vi "_ADC Calibration.vi"(0 "ADC In":string[][](table)) -> (1 "ADC Out":string[][](table), 2 "ADC Table":T1[](array[typedef]))   [LabVIEW 2012]
uses:
  Type/_RT Configuration 2.ctl
  Type/_RT Command.ctl
  Type/_RT Active Ch.ctl
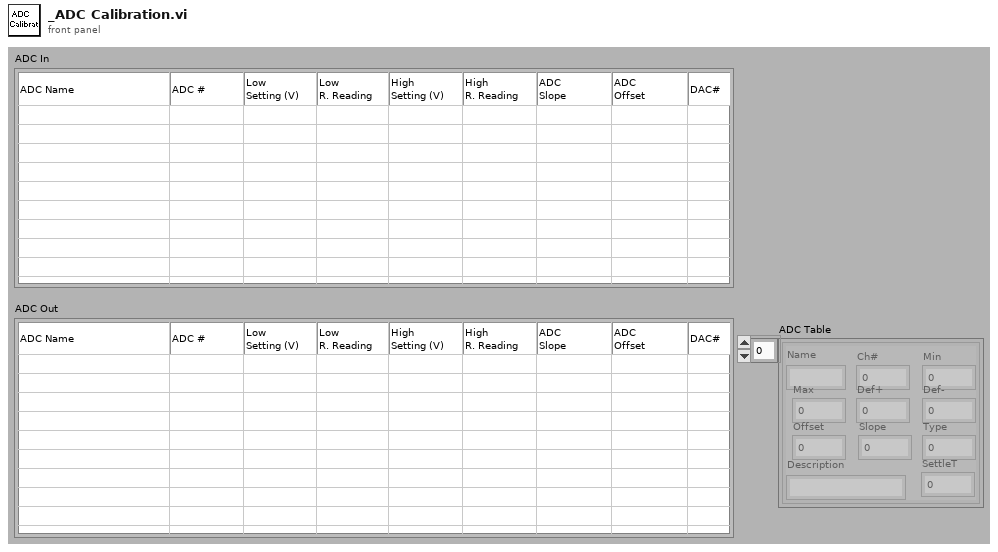
[diagram p1: front panel]
types:
  T1 = typedef "_RT Configuration 2.ctl" = cluster{"Name":string, "Ch#":u8, "Min":dbl, "Max":dbl, "Def+":dbl, "Def-":dbl, "Offset":dbl, "Slope":dbl, "Type":u8, "Description":string, "SettleT":dbl}
  T2 = typedef "_RT Command.ctl" = enum16{"Start", "Stop", "Runtime Update", "Get Data", "Get Info", "Get Status", "Get Param", "Get Config", "Get Table", "Read ADC", "Set Oscillator", "Update Config", "Update Table", "Set All Pol", "Set Pol and DC", "Set Max Mass", "Toggle RP", "Toggle EL", "Set PIC", "Initialize Turbo", "Send Turbo Comm", "Close Turbo", "P1", "P2", "P3", "Send Serial", "Set LC Out", "Get LC In", "Read VAC", "Test Table", "Toggle Power", "Get Startup", "Set Startup", "Get ADC Table", "Set ADC Table", "Get Brief Status", "Get Detail Status", "Auxiliary Update", "Set CC Logics", "Set CC Input Logics", "Ignore Error"}
  T3 = typedef "_RT Active Ch.ctl" = cluster{"Start":i32, "Step":i32, "ChID":i32}
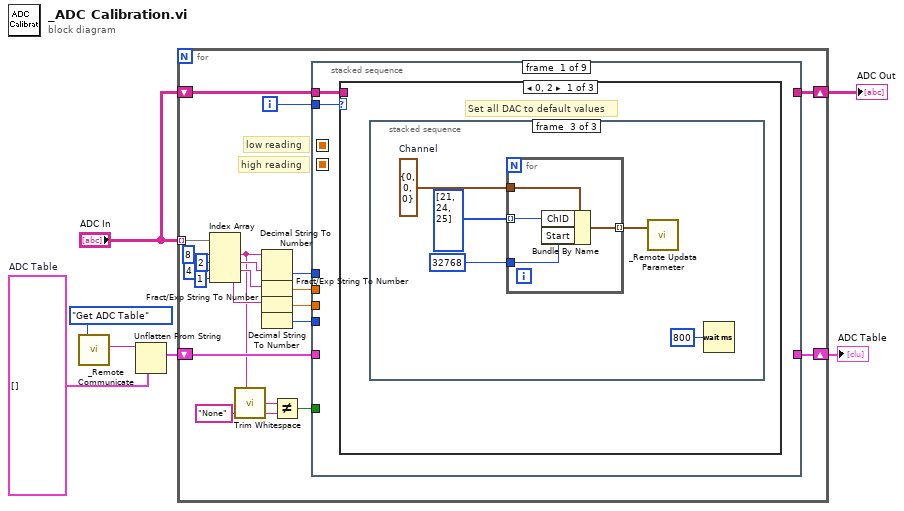
[diagram p0: block diagram]
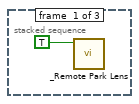
[diagram p2: hidden frame]
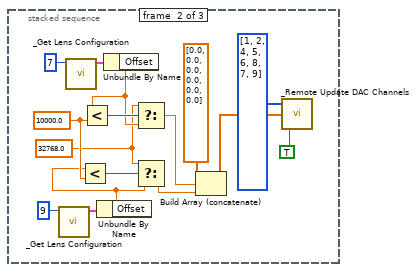
[diagram p3: hidden frame]
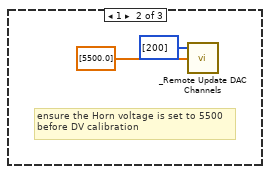
[diagram p4: hidden frame]
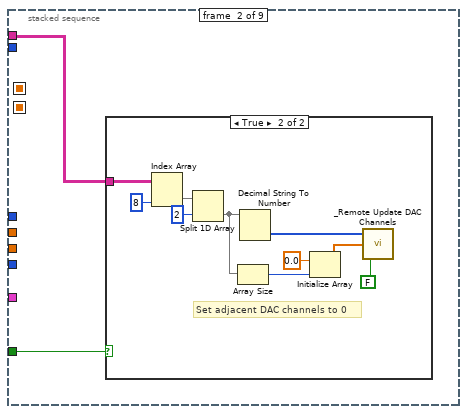
[diagram p6: hidden frame]
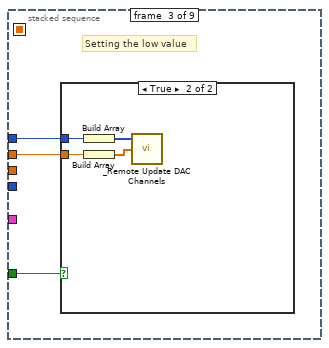
[diagram p8: hidden frame]
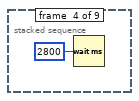
[diagram p10: hidden frame]
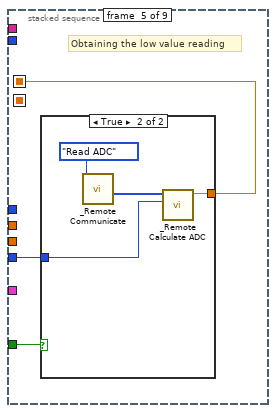
[diagram p11: hidden frame]
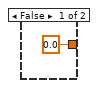
[diagram p12: hidden frame]
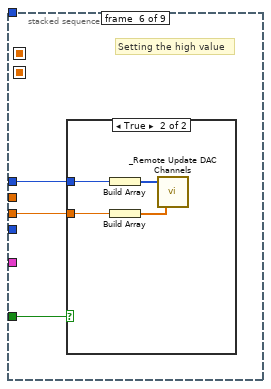
[diagram p13: hidden frame]
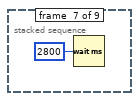
[diagram p15: hidden frame]
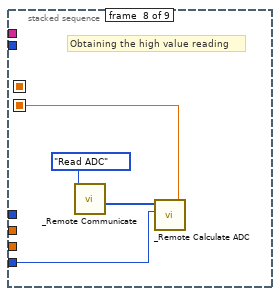
[diagram p16: hidden frame]
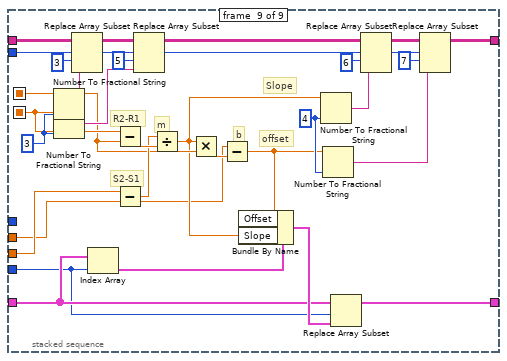
[diagram p17: hidden frame]
diagram:
  w3 = T1[] []  # ADC Table
  n1 = call "_Remote Communicate.vi"("Command"=_RT_Command."Get ADC Table") -> ("Info"=w4:string)  [unwired: 5 in, 3 out]
  n2 = Unflatten From String(type=w3, binary string=w4) -> (value=w2:T1[])  [unwired: 1 in, 4 out]
  n3 = for {
    tunnel: "ADC In" -> [w28] mode=indexing
    shift-right: [w22] -> w6
    shift-left: "ADC In" -> [w23]
    shift-right: [w12] -> w1
    shift-left: w2 -> [w21]
    i -> [w26]
    # "high reading"
    # "low reading"
    n4 = Index Array(array=w28, index #1=8 ("index"), index #2=2 ("index"), index #3=4 ("index"), index #4=1 ("index")) -> (element #1=w9:string, element #2=w19:string, element #3=w16:string, element #4=w14:string)
    n5 = call <vilib>:"Trim Whitespace.vi"("string"=w9) -> ("trimmed string"=w11:string)  [unwired: 1 in]
    n6 = Decimal String To Number(string=w9) -> (number=w27:i32)  [unwired: 3 out]
    n7 = Fract/Exp String To Number(string=w19) -> (number=w25:dbl)  [unwired: 4 out]
    n8 = Fract/Exp String To Number(string=w16) -> (number=w24:dbl)  [unwired: 4 out]
    n9 = Decimal String To Number(string=w14) -> (number=w13:i32)  [unwired: 3 out]
    n10 = Not Equal?(x=w11, y="None") -> (x != y?=w8:bool)
    n11 = stacked-sequence {
      seq-local: [_ _ _ _ w80 _ _ _ _] -> [_ _ _ _ _ _ _ _ w107]
      seq-local: [_ _ _ _ _ _ _ w95 _] -> [_ _ _ _ _ _ _ _ w111]
      tunnel: w27 -> [_ _ w73 _ _ w89 _ _ _]
      tunnel: w26 -> [w30 _ _ _ _ _ _ _ w115]
      tunnel: w25 -> [_ _ w72 _ _ _ _ _ w104]
      tunnel: w24 -> [_ _ _ _ _ w88 _ _ w110]
      tunnel: w23 -> [w29 w60 _ _ _ _ _ _ w117]
      tunnel: [_ _ _ _ _ _ _ _ w121] -> w22
      tunnel: w21 -> [_ _ _ _ _ _ _ _ w101]
      tunnel: w13 -> [_ _ _ _ w81 _ _ w96 w99]
      tunnel: [_ _ _ _ _ _ _ _ w100] -> w12
      tunnel: w8 -> [_ w59 w71 _ w79 w87 _ _ _]
      frame #0 {
        n12 = case shown="0, 2" w30 {
          tunnel: w29 -> [_ _ _]
          frame 0, 2 {
            # "Set all DAC to default values"
            n13 = stacked-sequence {
              frame #0 {
                n14 = call "_Remote Park Lens.vi"("All Ch (F)"=TRUE) -> ()  [unwired: 1 in, 6 out]
              }
              frame #1 {
                w36 = 32768.0 ("y")
                w38 = 10000.0 ("y")
                n15 = call "_Get Lens Configuration.vi"("Channel #"=u8 9) -> ("Lens Configuration"=w43:T1)  [unwired: 1 in, 5 out]
                n16 = call "_Get Lens Configuration.vi"("Channel #"=u8 7) -> ("Lens Configuration"=w44:T1)  [unwired: 1 in, 5 out]
                n17 = Unbundle By Name(w43) -> ("Offset"=w37:dbl)
                n18 = Less?(x=w37, y=w38) -> (x < y?=w39:bool)
                n19 = Unbundle By Name(w44) -> ("Offset"=w40:dbl)
                n20 = Less?(x=w40, y=w38) -> (x < y?=w41:bool)
                n21 = Select(t=w36, s=w41, f=w40) -> (s? t:f=w33:dbl)
                n22 = Select(t=w36, s=w39, f=w37) -> (s? t:f=w32:dbl)
                n23 = Build Array (concatenate)(dbl[] [0.0, 0.0, 0.0, 0.0, 0.0, 0.0] ("Ch#"), w33, w32) -> (w34:dbl[])
                n24 = call "_Remote Update DAC Channels.vi"("In DAC(F)"=TRUE ("Zero-DAC (F)"), "UserValue"=w34, "Ch#"=u8[] [1, 2, 4, 5, 6, 8, 7, 9]) -> ()  [unwired: 2 out]
              }
              frame #2 {
                w49 = T3 {"Start"=0, "Step"=0, "ChID"=0}  # Channel
                n25 = for {
                  tunnel: u8[] [21, 24, 25] ("Ch#") -> [w56] mode=indexing
                  tunnel: 32768 ("Start") -> [w55]
                  tunnel: w49 -> [w54]
                  tunnel: [w53] -> w48 mode=indexing
                  n26 = Bundle By Name(cluster=w54, "ChID"=w56, "Start"=w55) -> (w53:T3)
                }
                n27 = call "_Remote Updata Parameter.vi"("Parameters"=w48) -> ()  [unwired: 1 in, 1 out]
                n28 = Wait (ms)(milliseconds to wait=u32 800) -> ()  [unwired: 1 out]
              }
            }
          }
          frame 1 {
            # "ensure the Horn voltage is set to 5500\nbefore DV calibration"
            n29 = call "_Remote Update DAC Channels.vi"("UserValue"=dbl[] [5500.0], "Ch#"=i32[] [200]) -> ()  [unwired: 1 in, 2 out]
          }
          frame Default {
          }
        }
      }
      frame #1 {
        n30 = case shown="True" w59 {
          tunnel: w60 -> [_ w61]
          frame False {
          }
          frame True {
            # "Set adjacent DAC channels to 0"
            n31 = Index Array(array=w61, index (col)=8 ("disabled index (col)")) -> (element=w69:string[])  [unwired: 1 in]
            n32 = Split 1D Array(array=w69, index=2) -> (second subarray=w67:string[])  [unwired: 1 out]
            n33 = Array Size(array=w67) -> (size(s)=w66:i32)
            n34 = Decimal String To Number(string=w67) -> (number=w63:i32[])  [unwired: 3 out]
            n35 = Initialize Array(0.0 ("element"), w66) -> (w62:dbl[])
            n36 = call "_Remote Update DAC Channels.vi"("In DAC(F)"=FALSE ("Zero-DAC (F)"), "UserValue"=w62, "Ch#"=w63) -> ()  [unwired: 2 out]
          }
        }
      }
      frame #2 {
        # "Setting the low value"
        n37 = case shown="True" w71 {
          tunnel: w73 -> [_ w77]
          tunnel: w72 -> [_ w75]
          frame False {
          }
          frame True {
            n38 = Build Array(w77) -> (w76:i32[])
            n39 = Build Array(w75) -> (w74:dbl[])
            n40 = call "_Remote Update DAC Channels.vi"("UserValue"=w74, "Ch#"=w76) -> ()  [unwired: 1 in, 2 out]
          }
        }
      }
      frame #3 {
        n41 = Wait (ms)(milliseconds to wait=u32 2800) -> ()  [unwired: 1 out]
      }
      frame #4 {
        # "Obtaining the low value reading"
        n42 = case shown="True" w79 {
          tunnel: w81 -> [_ w84]
          tunnel: [0.0 ("Raw Reading") w83] -> w80
          frame False {
          }
          frame True {
            n43 = call "_Remote Communicate.vi"("Command"=_RT_Command."Read ADC") -> ("Data Array"=w85:i32[])  [unwired: 5 in, 3 out]
            n44 = call "_Remote Calculate ADC.vi"("ADC Channel (64)"=w84, "ADC Values"=w85) -> ("Raw Reading"=w83:dbl)  [unwired: 2 in, 3 out]
          }
        }
      }
      frame #5 {
        # "Setting the high value"
        n45 = case shown="True" w87 {
          tunnel: w89 -> [_ w93]
          tunnel: w88 -> [_ w90]
          frame False {
          }
          frame True {
            n46 = Build Array(w93) -> (w92:i32[])
            n47 = Build Array(w90) -> (w91:dbl[])
            n48 = call "_Remote Update DAC Channels.vi"("UserValue"=w91, "Ch#"=w92) -> ()  [unwired: 1 in, 2 out]
          }
        }
      }
      frame #6 {
        n49 = Wait (ms)(milliseconds to wait=u32 2800) -> ()  [unwired: 1 out]
      }
      frame #7 {
        # "Obtaining the high value reading"
        n50 = call "_Remote Communicate.vi"("Command"=_RT_Command."Read ADC") -> ("Data Array"=w97:i32[])  [unwired: 5 in, 3 out]
        n51 = call "_Remote Calculate ADC.vi"("ADC Channel (64)"=w96, "ADC Values"=w97) -> ("Raw Reading"=w95:dbl)  [unwired: 2 in, 3 out]
      }
      frame #8 {
        w114 = i16 3 ("precision (6)")
        w127 = i16 4 ("precision (6)")
        # "Slope"
        # "b"
        # "offset"
        # "m"
        # "S2-S1"
        # "R2-R1"
        n52 = Number To Fractional String(number=w107, precision (6)=w114) -> (F-format string=w113:string)  [unwired: 2 out]
        n53 = Number To Fractional String(number=w111, precision (6)=w114) -> (F-format string=w112:string)  [unwired: 2 out]
        n54 = Replace Array Subset(array=w117, new element=w113, index (row)=w115, index (col)=3 ("disabled index (col)")) -> (w120:string[][])
        n55 = Index Array(array=w101, index=w99) -> (element=w102:T1)
        n56 = Subtract(x=w111, y=w107) -> (x-y=w109:dbl)
        n57 = Subtract(x=w110, y=w104) -> (x-y=w108:dbl)
        n58 = Replace Array Subset(array=w120, new element=w112, index (row)=w115, index (col)=5 ("disabled index (col)")) -> (w116:string[][])
        n59 = Divide(x=w108, y=w109) -> (x/y=w106:dbl)
        n60 = Multiply(x=w106, y=w107) -> (x*y=w105:dbl)
        n61 = Subtract(x=w104, y=w105) -> (x-y=w103:dbl)
        n62 = Bundle By Name(cluster=w102, "Offset"=w103, "Slope"=w106) -> (w128:T1)
        n63 = Number To Fractional String(number=w106, precision (6)=w127) -> (F-format string=w125:string)  [unwired: 2 out]
        n64 = Number To Fractional String(number=w103, precision (6)=w127) -> (F-format string=w122:string)  [unwired: 2 out]
        n65 = Replace Array Subset(array=w101, new element=w128, index=w99) -> (w100:T1[])
        n66 = Replace Array Subset(array=w116, new element=w125, index (row)=w115, index (col)=6 ("disabled index (col)")) -> (w123:string[][])
        n67 = Replace Array Subset(array=w123, new element=w122, index (row)=w115, index (col)=7 ("disabled index (col)")) -> (w121:string[][])
      }
    }
  }
  "ADC Out" <- w6
  "ADC Table" <- w1
